vi "from string 1.0.vi"(8 "error in (no error)":errorcluster, 10 "data":string, 11 "Formatter Config in":refnum<class "Formatter Config.lvclass">) -> (0 "error out":errorcluster, 3 "Formatter Config out":refnum<class "Formatter Config.lvclass">)   [LabVIEW 2015, in "Formatter Config.lvclass"]
uses:
  Formatter Config.lvclass
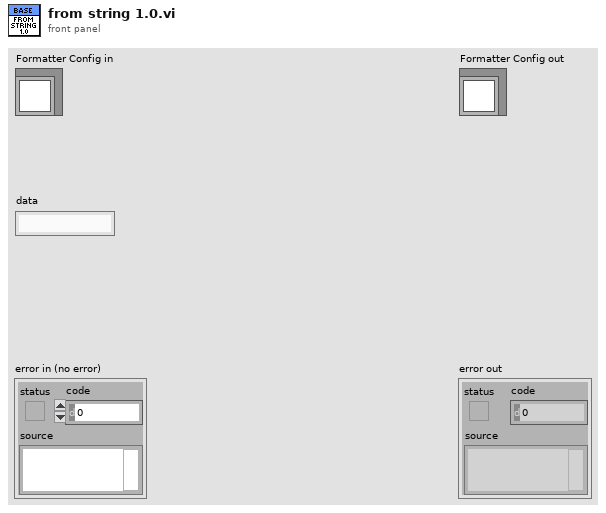
[diagram p1: front panel]
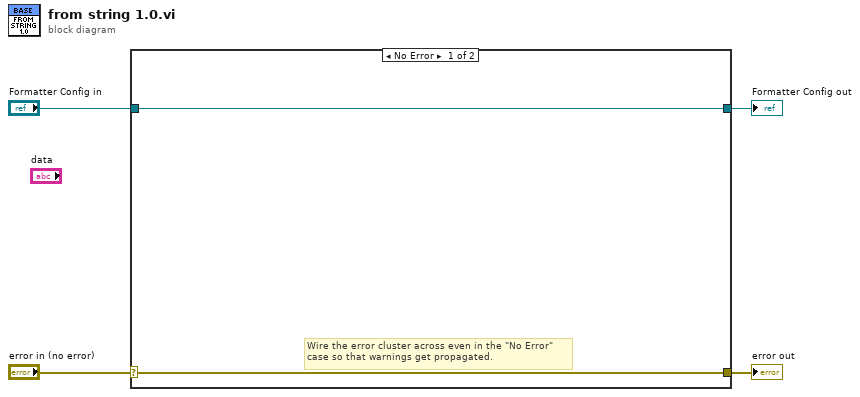
[diagram p0: block diagram]
diagram:
  n1 = case shown="No Error" "error in (no error)" {
    selector: "error in (no error)" -> [w5 w8]
    tunnel: [w5 w8] -> w3
    tunnel: [w6 w7] -> w1
    tunnel: "Formatter Config in" -> [w6 w7]
    frame No Error {
      # "Wire the error cluster across even in the \"No Error\"\ncase so that warnings get propagated."
    }
    frame Error {
    }
  }
  "error out" <- w3
  "Formatter Config out" <- w1
